vi "Set Position.vi"(8 "error in (no error)":errorcluster, 10 "Positions":T1, 11 "VI in":refnum<vi>) -> (0 "error out":errorcluster)   [LabVIEW 2014, in "Chart Module.lvlib"]
uses:
  Chart Module.lvlib
  Position--enum.ctl
  <vilib>/Utility/miscctls.llb/LVRectTypeDef.ctl
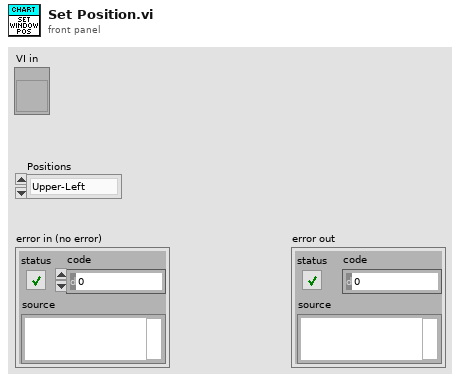
[diagram p1: front panel]
types:
  T1 = typedef "Chart Module.lvlib/Position--enum.ctl" = enum16{"Upper-Left", "Upper-Center", "Upper-Right", "Center-left", "Center", "Center-Right", "Bottom-Left", "Bottom-Center", "Bottom-Right", ""}
  T2 = typedef "LVRectTypeDef.ctl" = cluster{"Left":i16, "Top":i16, "Right":i16, "Bottom":i16}
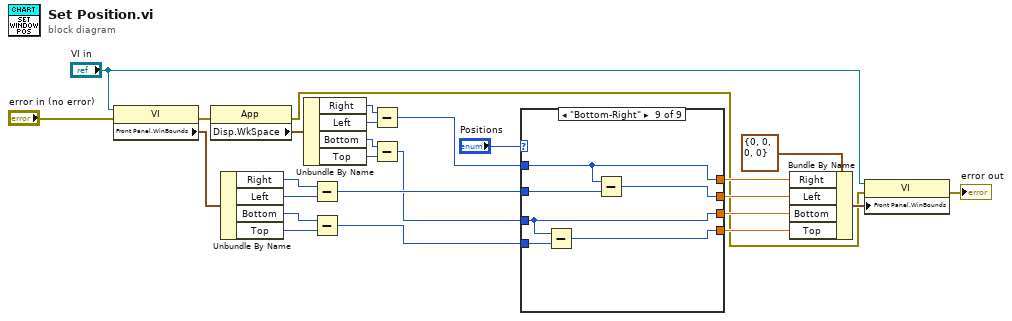
[diagram p0: block diagram]
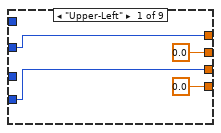
[diagram p2: hidden frame]
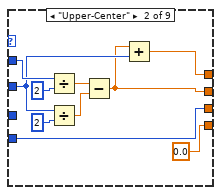
[diagram p3: hidden frame]
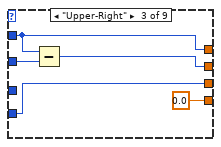
[diagram p4: hidden frame]
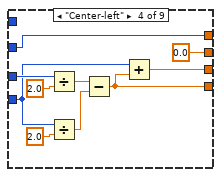
[diagram p5: hidden frame]
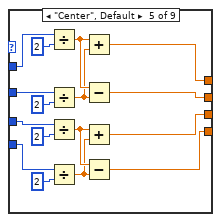
[diagram p6: hidden frame]
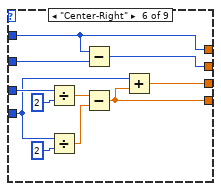
[diagram p7: hidden frame]
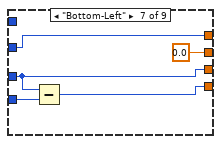
[diagram p8: hidden frame]
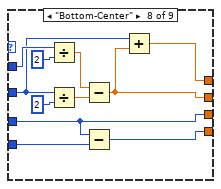
[diagram p9: hidden frame]
diagram:
  n1 = property class="VI"(reference="VI in", error in="error in (no error)") -> (error out=w3:errorcluster, "Front Panel.WinBounds"=w13:T2)  [unwired: 1 out]
  n2 = property class="App"(error in=w3) -> (error out=w1:errorcluster, "Disp.WkSpace"=w22:T2)  [unwired: 1 in, 1 out]
  n3 = Unbundle By Name(w13) -> ("Right"=w14:i16, "Left"=w15:i16, "Bottom"=w16:i16, "Top"=w17:i16)
  n4 = Unbundle By Name(w22) -> ("Right"=w21:i16, "Left"=w20:i16, "Bottom"=w19:i16, "Top"=w18:i16)
  n5 = Subtract(x=w14, y=w15) -> (x-y=w25:i16)
  n6 = Subtract(x=w16, y=w17) -> (x-y=w26:i16)
  n7 = Subtract(x=w21, y=w20) -> (x-y=w23:i16)
  n8 = Subtract(x=w19, y=w18) -> (x-y=w24:i16)
  n9 = case shown="\"Bottom-Right\"" "Positions" {
    tunnel: [w29 w33 w45 w54 w67 w82 w86 w88 w104] -> w8
    tunnel: [0.0 w31 w43 0.0 w66 w80 0.0 w90 w102] -> w9
    tunnel: [0.0 0.0 0.0 w48 w65 w74 w84 w97 w101] -> w11
    tunnel: [w27 w39 w41 w46 w64 w72 w85 w98 w100] -> w10
    tunnel: w23 -> [_ w38 w45 _ w60 w82 _ w95 w104]
    tunnel: w24 -> [_ _ _ w53 w58 w79 w85 w98 w100]
    tunnel: w25 -> [w29 w32 w44 w54 w57 w81 w86 w89 w103]
    tunnel: w26 -> [w27 w39 w41 w47 w56 w73 w83 w96 w99]
    frame "Upper-Left" {
    }
    frame "Upper-Center" {
      n10 = Divide(x=w38, y=i16 2) -> (x/y=w35:dbl)
      n11 = Divide(x=w32, y=i16 2) -> (x/y=w34:dbl)
      n12 = Subtract(x=w35, y=w34) -> (x-y=w31:dbl)
      n13 = Add(x=w31, y=w32) -> (x+y=w33:dbl)
    }
    frame "Upper-Right" {
      n14 = Subtract(x=w45, y=w44) -> (x-y=w43:i16)
    }
    frame "Center-left" {
      n15 = Divide(x=w53, y=2.0) -> (x/y=w50:dbl)
      n16 = Divide(x=w47, y=2.0) -> (x/y=w49:dbl)
      n17 = Subtract(x=w50, y=w49) -> (x-y=w48:dbl)
      n18 = Add(x=w47, y=w48) -> (x+y=w46:dbl)
    }
    frame "Center", Default {
      n19 = Divide(x=w60, y=i16 2) -> (x/y=w71:dbl)
      n20 = Divide(x=w57, y=i16 2) -> (x/y=w70:dbl)
      n21 = Divide(x=w58, y=i16 2) -> (x/y=w69:dbl)
      n22 = Divide(x=w56, y=i16 2) -> (x/y=w68:dbl)
      n23 = Add(x=w71, y=w70) -> (x+y=w67:dbl)
      n24 = Subtract(x=w71, y=w70) -> (x-y=w66:dbl)
      n25 = Add(x=w69, y=w68) -> (x+y=w64:dbl)
      n26 = Subtract(x=w69, y=w68) -> (x-y=w65:dbl)
    }
    frame "Center-Right" {
      n27 = Divide(x=w79, y=i16 2) -> (x/y=w76:dbl)
      n28 = Divide(x=w73, y=i16 2) -> (x/y=w75:dbl)
      n29 = Subtract(x=w82, y=w81) -> (x-y=w80:i16)
      n30 = Subtract(x=w76, y=w75) -> (x-y=w74:dbl)
      n31 = Add(x=w73, y=w74) -> (x+y=w72:dbl)
    }
    frame "Bottom-Left" {
      n32 = Subtract(x=w85, y=w83) -> (x-y=w84:i16)
    }
    frame "Bottom-Center" {
      n33 = Divide(x=w95, y=i16 2) -> (x/y=w92:dbl)
      n34 = Divide(x=w89, y=i16 2) -> (x/y=w91:dbl)
      n35 = Subtract(x=w92, y=w91) -> (x-y=w90:dbl)
      n36 = Subtract(x=w98, y=w96) -> (x-y=w97:i16)
      n37 = Add(x=w89, y=w90) -> (x+y=w88:dbl)
    }
    frame "Bottom-Right" {
      n38 = Subtract(x=w100, y=w99) -> (x-y=w101:i16)
      n39 = Subtract(x=w104, y=w103) -> (x-y=w102:i16)
    }
  }
  n40 = Bundle By Name(cluster=T2 {"Left"=0, "Top"=0, "Right"=0, "Bottom"=0} ("Front Panel Window:Window Bounds"), "Right"=w8, "Left"=w9, "Bottom"=w10, "Top"=w11) -> (w12:T2)
  n41 = property class="VI"(reference="VI in", error in=w1, "Front Panel.WinBounds"=w12) -> (error out=→"error out":errorcluster)  [unwired: 1 out]
